vi "Smooth Background CDBL.vi"(7 "Type":T1(ring)=enum."Bandpass", 8 "Error In":errorcluster, 9 "HP F":dbl format="%#_6p", 10 "LP  F":dbl=0.001 format="%#_6p", 11 "Data":cdb[](array[numeric])) -> (0 "Error Out":errorcluster, 3 "Data out":cdb[](array[numeric]))   [LabVIEW 2016]
uses:
  <vilib>/measure/NI_MAPro.lvlib
  <vilib>/measure/macond.llb/IIR Filter for 1 Chan (CDB).vi
  <vilib>/Analysis/3filter.llb/Filter Structure Type.ctl
  <vilib>/Analysis/NI_AALBase.lvlib
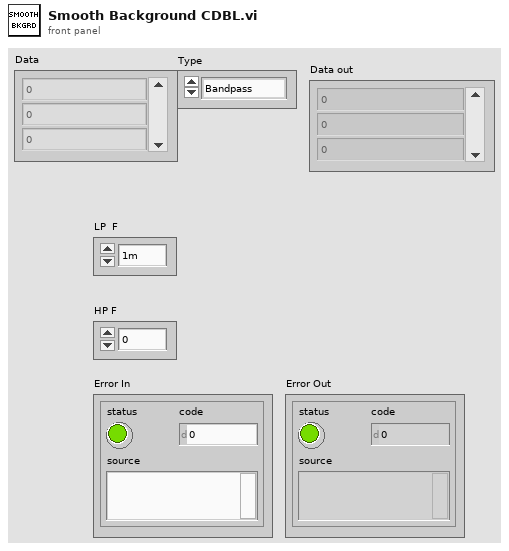
[diagram p1: front panel]
types:
  T1 = enum16{"Lowpass", "Highpass", "Bandpass", "Bandstop"}
  T2 = typedef "NI_AALBase.lvlib/Filter Structure Type.ctl" = u16
  T3 = cluster{"Topology":enum16{"Off", "Butterworth", "Chebyshev", "Inverse Chebyshev", "Elliptic", "Bessel"}, "Type":enum16{"Lowpass", "Highpass", "Bandpass", "Bandstop"}, "Order":i32, "Lower Fc":dbl, "Upper Fc":dbl, "PB Ripple":dbl, "SB Attenuation":dbl}
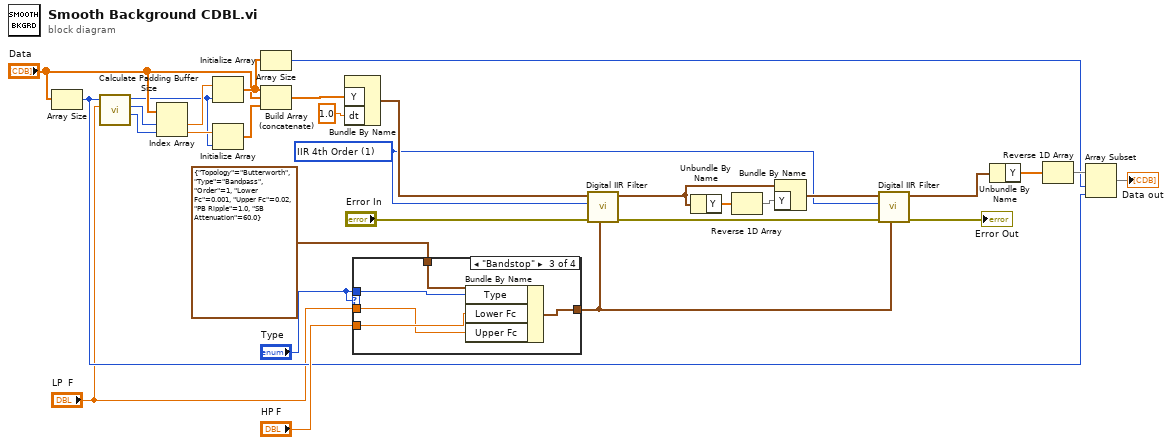
[diagram p0: block diagram]
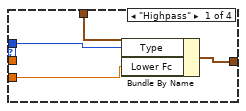
[diagram p2: hidden frame]
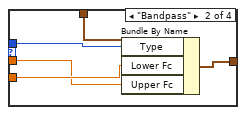
[diagram p3: hidden frame]
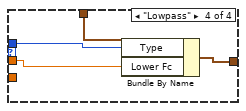
[diagram p4: hidden frame]
diagram:
  w18 = T2 1 items=["IIR 2nd Order"=0, "IIR 4th Order"=1, "Auto Select"=10] ("filter structure option")
  n1 = Array Size(array="Data") -> (size(s)=w6:i32)
  n2 = call "Calculate Padding Buffer Size.vi"("LP  F"="LP  F", "Array size"=w6) -> ("Last element"=w2:i32, "First element"=w3:i32, "Buffer size"=w4:i32)  [unwired: 7 in]
  n3 = Index Array(array="Data", index #1=w3, index #2=w2) -> (element #1=w28:cdb, element #2=w10:cdb)
  n4 = Initialize Array(w28, w4) -> (w30:cdb[])
  n5 = Initialize Array(w10, w4) -> (w9:cdb[])
  n6 = Array Size(array=w30) -> (size(s)=w13:i32)
  n7 = Build Array (concatenate)(w30, "Data", w9) -> (w29:cdb[])
  n8 = Bundle By Name("Y"=w29, "dt"=1.0) -> (w26:waveform(cdb))  [unwired: 1 in]
  n9 = case shown="\"Bandstop\"" "Type" {
    tunnel: T3 {"Topology"=enum."Butterworth", "Type"=enum."Bandpass", "Order"=1, "Lower Fc"=0.001, "Upper Fc"=0.02, "PB Ripple"=1.0, "SB Attenuation"=60.0} ("IIR filter specifications") -> [w34 w39 w44 w48]
    tunnel: "HP F" -> [w31 w36 w41 _]
    tunnel: [w33 w38 w43 w47] -> w19
    tunnel: "Type" -> [w32 w37 w42 w46]
    tunnel: "LP  F" -> [_ w35 w40 w45]
    frame "Highpass" {
      n10 = Bundle By Name(cluster=w34, "Type"=w32, "Lower Fc"=w31) -> (w33:T3)
    }
    frame "Bandpass" {
      n11 = Bundle By Name(cluster=w39, "Type"=w37, "Lower Fc"=w36, "Upper Fc"=w35) -> (w38:T3)
    }
    frame "Bandstop" {
      n12 = Bundle By Name(cluster=w44, "Type"=w42, "Lower Fc"=w41, "Upper Fc"=w40) -> (w43:T3)
    }
    frame "Lowpass" {
      n13 = Bundle By Name(cluster=w48, "Type"=w46, "Lower Fc"=w45) -> (w47:T3)
    }
  }
  n14 = call-poly <vilib>:"Digital IIR Filter.vi"("IIR filter specifications"=w19, "error in (no error)"="Error In", "filter structure option"=w18, "signal in"=w26) -> ("error out"=w17:errorcluster, "signal out"=w22:waveform(cdb))  [unwired: 5 in, 1 out]
  n15 = Unbundle By Name(w22) -> ("Y"=w23:cdb[])
  n16 = Reverse 1D Array(array=w23) -> (reversed array=w21:cdb[])
  n17 = Bundle By Name(cluster=w22, "Y"=w21) -> (w20:waveform(cdb))
  n18 = call-poly <vilib>:"Digital IIR Filter.vi"("IIR filter specifications"=w19, "error in (no error)"=w17, "filter structure option"=w18, "signal in"=w20) -> ("error out"=→"Error Out":errorcluster, "signal out"=w15:waveform(cdb))  [unwired: 5 in, 1 out]
  n19 = Unbundle By Name(w15) -> ("Y"=w16:cdb[])
  n20 = Reverse 1D Array(array=w16) -> (reversed array=w14:cdb[])
  n21 = Array Subset(array=w14, index=w13, length=w6) -> (→"Data out":cdb[])
